vi "Voice_Amp_Check.vi"(8 "error in (no error)":errorcluster, 11 "IN":T1={"step name 1"="", "updata 2"="0.22", "limitdata 3"="0.101", "load vi name 4"="", "parameter 5"=""}) -> (0 "error out":errorcluster, 3 "Cluster":T2)   [LabVIEW 2013]
uses:
  <vilib>/sound2/lvsound2.llb/Sampling Mode.ctl
  <vilib>/sound2/lvsound2.llb/Sound Data Format.ctl
  <vilib>/sound2/lvsound2.llb/Sound Input Read (DBL).vi
  <vilib>/measure/matone.llb/Extract Single Tone Information N Chan.vi
  <vilib>/measure/NI_MAPro.lvlib
panel:
  # "Hi: 750~0.22"
  # "Lo: 650~0.101"
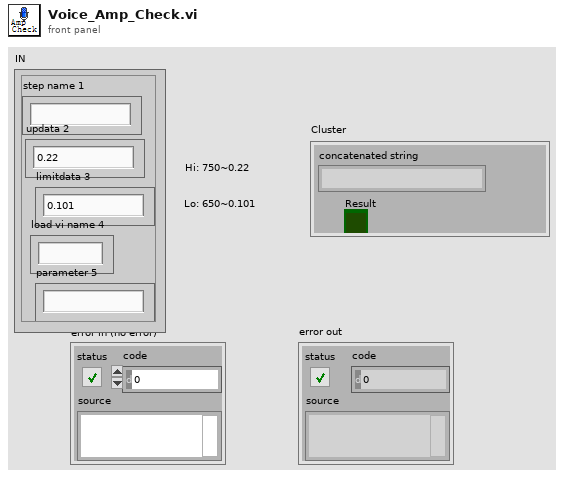
[diagram p1: front panel]
types:
  T1 = cluster{"step name 1":string, "updata 2":string, "limitdata 3":string, "load vi name 4":string, "parameter 5":string}
  T2 = cluster{"concatenated string":string, "Result":bool}
  T3 = typedef "Sound Data Format.ctl" = cluster{"sample rate (S/s)":dbl, "number of channels":i32, "bits per sample":i32}
  T4 = typedef "Sampling Mode.ctl" = i32
  T5 = typedef "Sound Input Task ID.ctl" = u32
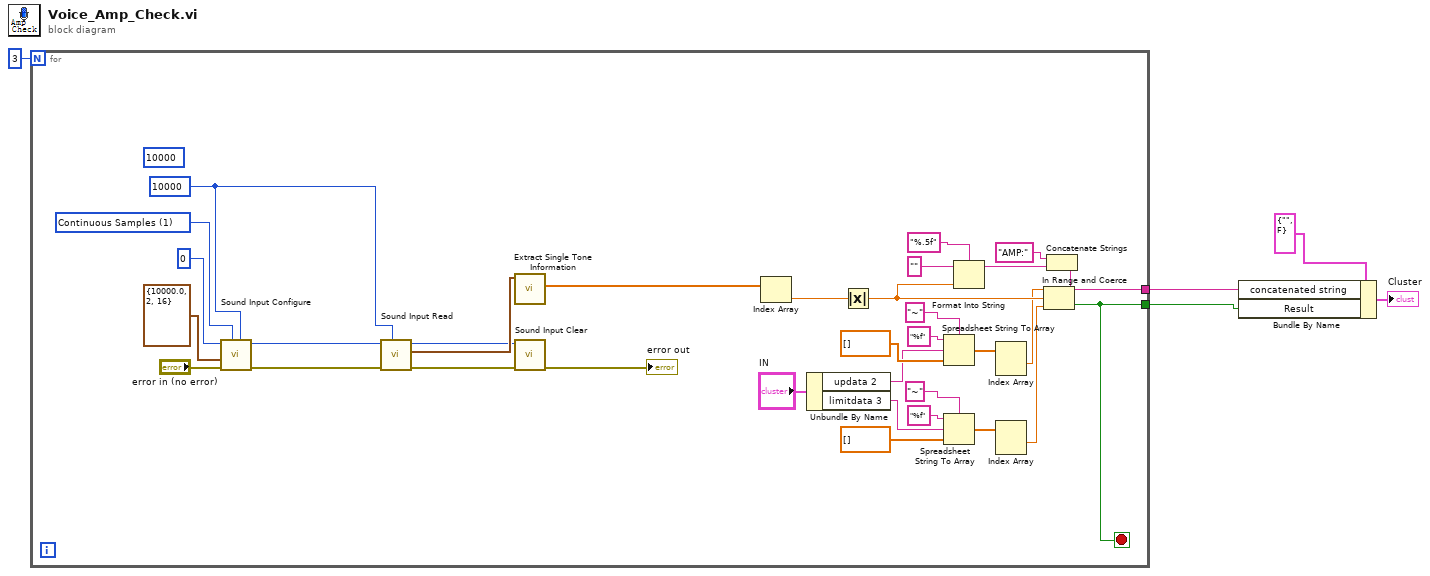
[diagram p0: block diagram]
diagram:
  n1 = for {
    N: 3 -> [_]
    tunnel: [w19] -> w3
    tunnel: [w6] -> w2
    stop <- w6 stop-if-true
    (unwired) 10000 ("Number of Samples/ch")
    w33 = 10000 ("Number of Samples/ch")
    w32 = T4 1 items=["Finite Samples", "Continuous Samples"] ("sample mode")
    n2 = call <vilib>:"Sound Input Configure.vi"("number of samples/ch"=w33, "sample mode"=w32, "error in (no error)"="error in (no error)", "sound format"=T3 {"sample rate (S/s)"=10000.0, "number of channels"=2, "bits per sample"=16} ("Sound Format"), "device ID"=u32 0 ("Device ID")) -> ("error out"=w27:errorcluster, "task ID"=w29:T5)  [unwired: 2 in, 3 out]
    n3 = call-poly <vilib>:"Sound Input Read.vi"("number of samples/ch"=w33, "error in (no error)"=w27, "task ID"=w29) -> ("error out"=w31:errorcluster, "data"=w36:waveform(dbl)[], "task ID out"=w30:T5)  [unwired: 1 in, 5 out]
    n4 = call-poly <vilib>:"Extract Single Tone Information.vi"("time signals in"=w36) -> ("detected amplitudes"=w35:dbl[])  [unwired: 3 in, 7 out]
    n5 = call <vilib>:"Sound Input Clear.vi"("error in (no error)"=w31, "task ID"=w30) -> ("error out"=→"error out":errorcluster)  [unwired: 9 out]
    n6 = Index Array(array=w35) -> (element=w37:dbl)  [unwired: 1 in]
    n7 = Unbundle By Name("IN") -> ("updata 2"=w16:string, "limitdata 3"=w11:string)
    n8 = Absolute Value(x=w37) -> (abs(x)=w20:dbl)
    n9 = Spreadsheet String To Array(delimiter (Tab)="~", format string="%f", spreadsheet string=w16, array type (2D Dbl)=dbl[] []) -> (array=w10:dbl[])
    n10 = Spreadsheet String To Array(delimiter (Tab)="~", format string="%f", spreadsheet string=w11, array type (2D Dbl)=dbl[] []) -> (array=w9:dbl[])
    n11 = Format Into String(format string="%.5f", initial string="", w20) -> (resulting string=w23:string)  [unwired: 1 in, 1 out]
    n12 = Index Array(array=w10) -> (element #1=w8:dbl)  [unwired: 2 in, 1 out]
    n13 = Index Array(array=w9) -> (element #1=w7:dbl)  [unwired: 2 in, 1 out]
    n14 = In Range and Coerce(upper limit=w8, x=w20, lower limit=w7) -> (In Range?=w6:bool)  [unwired: 1 out]
    n15 = Concatenate Strings("AMP:" ("string"), w23) -> (w19:string)
  }
  n16 = Bundle By Name(cluster=T2 {"concatenated string"="", "Result"=FALSE} ("Cluster"), "concatenated string"=w3, "Result"=w2) -> (→"Cluster":T2)
